vi "OPCUA InitTagGroup.vi"(8 "error in (no error)":errorcluster, 10 "publish interval (ms)":i32, 11 "reference":refnum<k24>) -> (0 "error out":errorcluster, 3 "reference 2":refnum<k24>)   [LabVIEW 2019]
uses:
  F:/src/HUTCDLSVN/Machine/CDL0100/TagEngine/LVOPCUA.NET/LVOPC.NETInterface/bin/Release/LVOPC.NETInterface.dll
  LVOPCUA.NET/LVOPC.NETInterface/bin/Release/LVOPC.NETInterface.dll
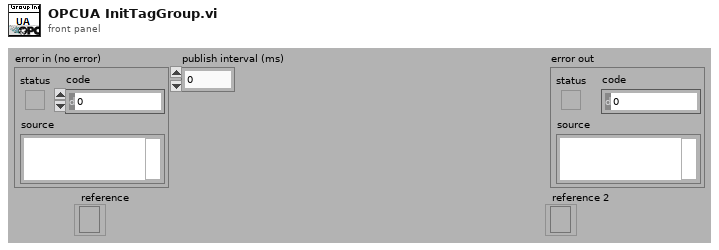
[diagram p1: front panel]
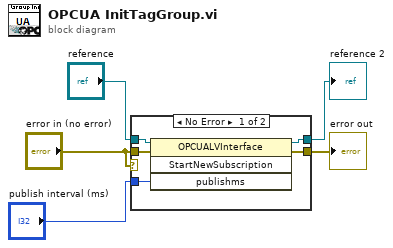
[diagram p0: block diagram]
diagram:
  n1 = case shown="No Error" "error in (no error)" {
    selector: "error in (no error)" -> [_ w12]
    tunnel: "error in (no error)" -> [w9 _]
    tunnel: [w8 w12] -> w5
    tunnel: "reference" -> [w10 w11]
    tunnel: [w7 w11] -> w2
    tunnel: "publish interval (ms)" -> [w6 _]
    frame No Error {
      n2 = invoke class="OPCUALVInterface" method="StartNewSubscription"(reference=w10, error in=w9, "publishms"=w6) -> (reference out=w7:refnum<k24>, error out=w8:errorcluster)  [unwired: 1 in, 2 out]
    }
    frame Error {
    }
  }
  "error out" <- w5
  "reference 2" <- w2
